vi "practiceImageAnalysis20vi.vi"() -> ()   [LabVIEW 2016]
uses:
  <vilib>/vision/Measure.llb/Straight Edge Options.ctl
  <vilib>/vision/Measure.llb/Straight Edge Process.ctl
  <vilib>/vision/Measure.llb/Edge Options.ctl
  <vilib>/vision/Measure.llb/Edge Polarity.ctl
  <vilib>/Analysis/6fits.llb/Curve Fitting Criteria.ctl
  <vilib>/Utility/file.llb/Write Delimited Spreadsheet (DBL).vi
  <vilib>/regexp/Match Regular Expression.xnode
  <vilib>/Analysis/NI_AALPro.lvlib
panel:
  in  "x values for fit line on plot":dbl[](array[numeric])=[-700.0, -300.0, 100.0, 500.0, 700.0]
  out "Bottom intercept":dbl
  out "Bottom slope":dbl
  out "Top intercept":dbl
  in  "method":T1 items=["Least Square", "Least Absolute Residual", "Bisquare"]
  out "Top slope":dbl
  out "Each point on located edges":T2(graph)
  out "Coordinate array for image capture":dbl[][](array[numeric])
  in  "Coordinate file for image capture":path=path "E:/XYZstage+Camera_CollectedImages/12-16-2016/noStaveMount/toolingpinsCoordinates-captured.csv"
  out "Review":bool
  out "Search running?":bool
  in  "Options: Bottom Edge Search":T5={"Search Direction"=3, "Edge Options"={"Edge Polarity"=2, "Kernel Size"=9, "Width"=3, "Minimum Edge Strength"=17.0, "Interpolation Type"=enum."Bilinear Fixed", "Data Processing Method"=enum."Average"}, "Show Search Area"=TRUE, "Show Search Lines"=TRUE, "Show Edges Found"=TRUE, "Show Result"=TRUE, "Search Area Color"=65280, "Search Lines Color"=255, "Edge Locations Color"=16776960, "Result Color"=16711680, "Overlay Group Name"=""} {"Search Direction" items=["Left to Right", "Right to Left", "Top to Bottom", "Bottom to Top"]; "Edge Options"."Edge Polarity" items=["All Edges", "Rising Edges", "Falling Edges"]; "Edge Options"."Minimum Edge Strength" format="%.2f"; "Edge Options"."Width" step=2; "Edge Options"."Kernel Size" step=2}
  in  "Options: Top Edge Search":T5={"Search Direction"=2, "Edge Options"={"Edge Polarity"=0, "Kernel Size"=5, "Width"=3, "Minimum Edge Strength"=16.0, "Interpolation Type"=enum."Bilinear Fixed", "Data Processing Method"=enum."Average"}, "Show Search Area"=TRUE, "Show Search Lines"=TRUE, "Show Edges Found"=TRUE, "Show Result"=TRUE, "Search Area Color"=65280, "Search Lines Color"=255, "Edge Locations Color"=16776960, "Result Color"=16711680, "Overlay Group Name"=""} {"Search Direction" items=["Left to Right", "Right to Left", "Top to Bottom", "Bottom to Top"]; "Edge Options"."Edge Polarity" items=["All Edges", "Rising Edges", "Falling Edges"]; "Edge Options"."Minimum Edge Strength" format="%.2f"; "Edge Options"."Width" step=2; "Edge Options"."Kernel Size" step=2}
  in  "Fit Options":T6={"Number of Lines"=1, "Type"=enum."First Edge Rake", "Min. Score"=10.0, "Max. Score"=1000.0, "Orientation"=0.0, "Angle Range"=45.0, "Angle Tolerance"=1.0, "Step Size"=196, "Min. SNR (db)"=0.0, "Min. Points (%)"=25.0, "Hough Iterations"=5} {"Min. Points (%)" min=0.0 max=100.0; "Min. SNR (db)" min=0.0; "Max. Score" min=0.0 max=1024.0; "Min. Score" min=0.0 max=1024.0 step=1.0}
  in  "Stop and delete":bool
  out "Images Array":T8[](array[plugin-control])
  in  "error in":errorcluster
  out "error out":errorcluster
  out "Filenames Array":string[](array[string])
  in  "Naming Convention":string="*.png"
  in  "Images Directory":path=path "E:/XYZstage+Camera_CollectedImages/12-16-2016/noStaveMount/toolingpins_images"
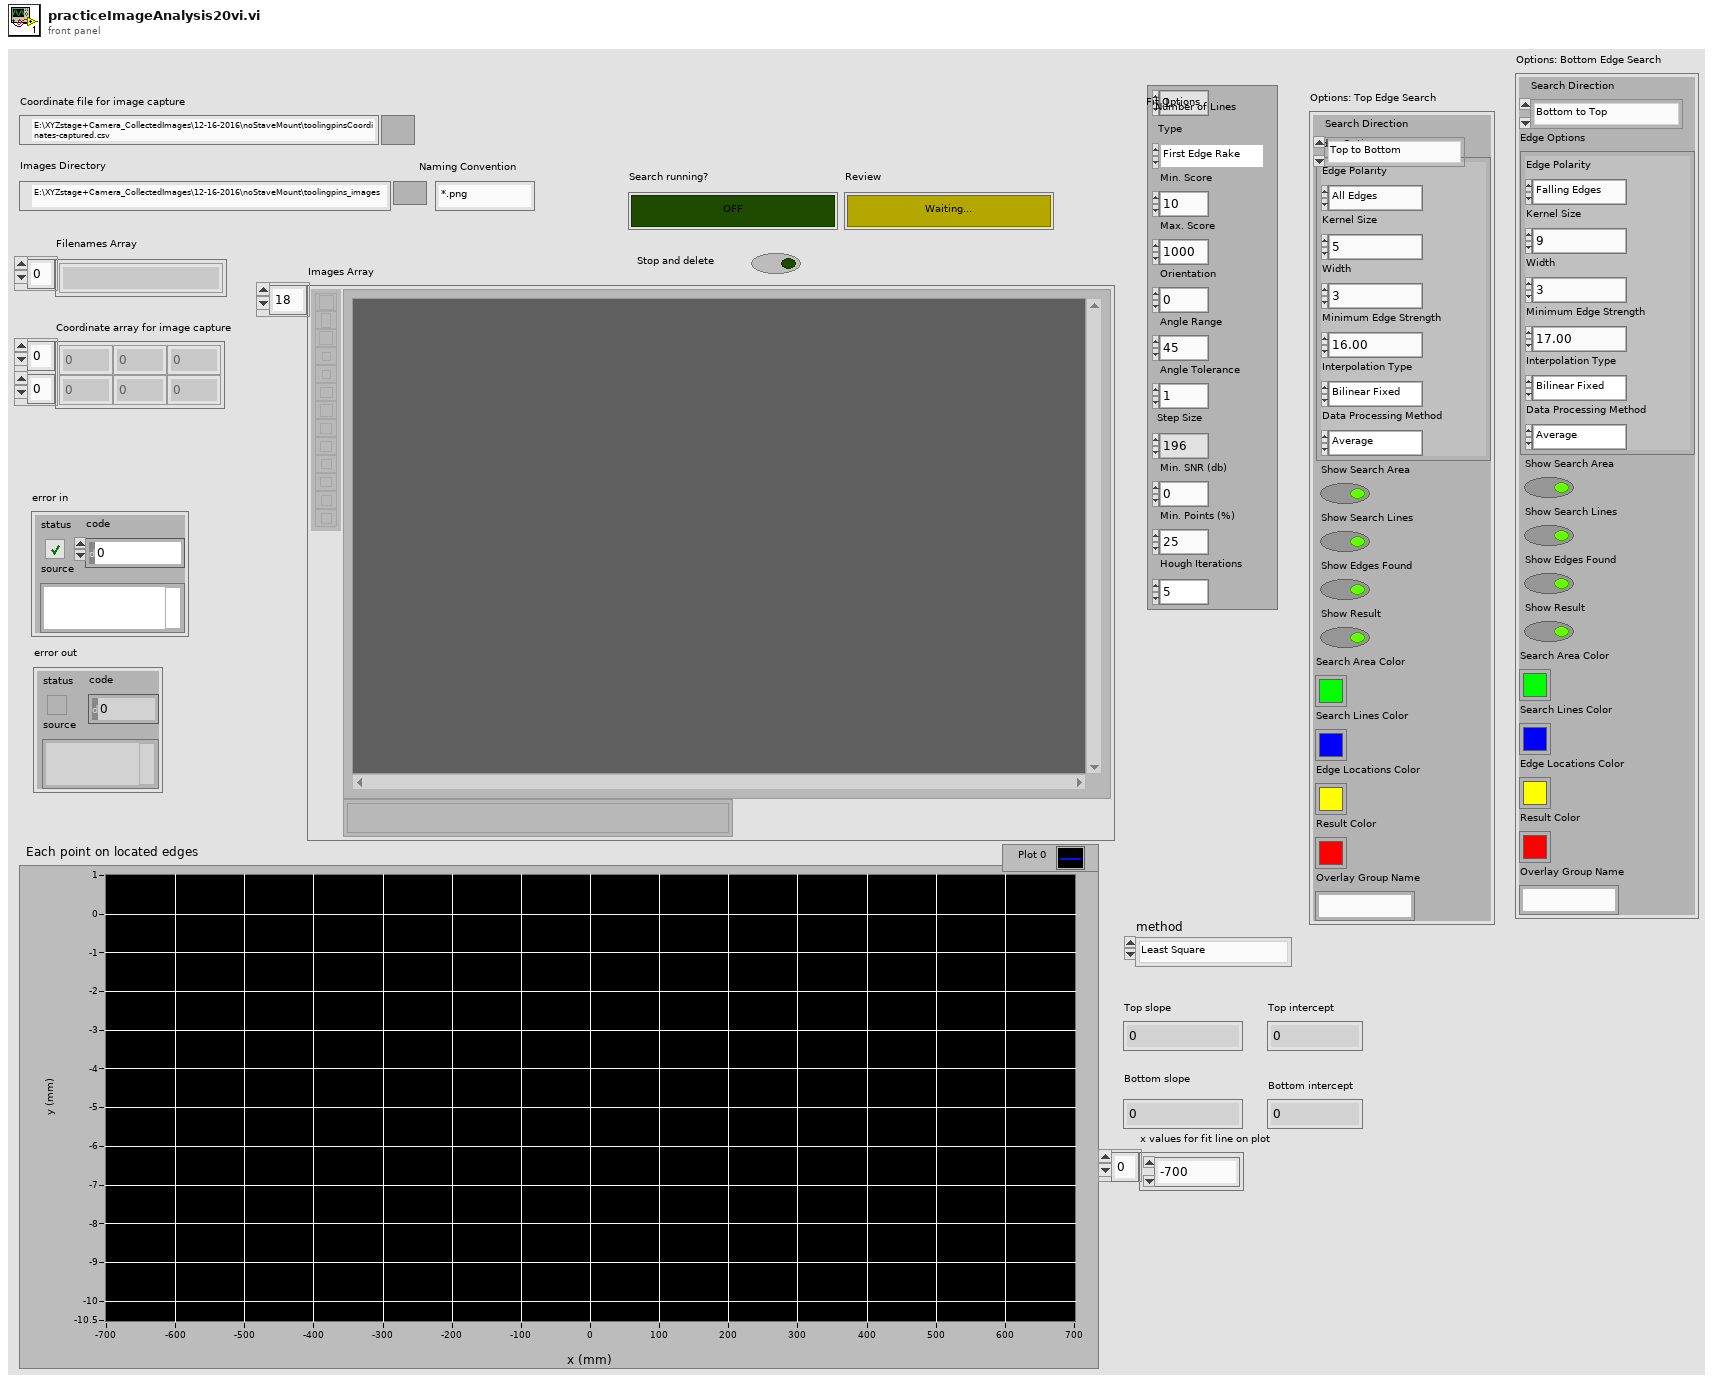
[diagram p1: front panel]
types:
  T1 = typedef "NI_AALPro.lvlib/Curve Fitting Criteria.ctl" = u16
  T2 = cluster{"Top averages":dbl[], "Best Linear Fit":dbl[]}[]
  T3 = typedef "Edge Options.ctl" = cluster{"Edge Polarity":T4, "Kernel Size":u32, "Width":u32, "Minimum Edge Strength":sgl, "Interpolation Type":enum32{"Zero Order", "Bilinear", "Quadratic", "Cubic", "Bilinear Fixed"}, "Data Processing Method":enum32{"Average", "Median"}}
  T4 = typedef "Edge Polarity.ctl" = u32
  T5 = cluster{"Search Direction":u32, "Edge Options":T3, "Show Search Area":bool, "Show Search Lines":bool, "Show Edges Found":bool, "Show Result":bool, "Search Area Color":u32, "Search Lines Color":u32, "Edge Locations Color":u32, "Result Color":u32, "Overlay Group Name":string}
  T6 = typedef "Straight Edge Options.ctl" = cluster{"Number of Lines":i32, "Type":T7, "Min. Score":dbl, "Max. Score":dbl, "Orientation":dbl, "Angle Range":dbl, "Angle Tolerance":dbl, "Step Size":u32, "Min. SNR (db)":dbl, "Min. Points (%)":dbl, "Hough Iterations":i32}
  T7 = typedef "Straight Edge Process.ctl" = enum32{"First Edge Rake", "Best Edge Rake", "Hough Edge Rake", "First Edge Projection", "Best Edge Projection"}
  T8 = typedef "IMAQ Image.ctl" = refnum<image>
  T9 = enum16{"cm", "mm", "pixels [mm/pix]", "pixels [um/pix]"}
  T10 = cluster{"Top averages":dbl[], "Top averages":dbl[]}
  T11 = cluster{"x values for fit line on plot":dbl[], "Array":dbl[]}
  T12 = cluster{"x values for fit line on plot":dbl[], "Array":dbl[]}[]
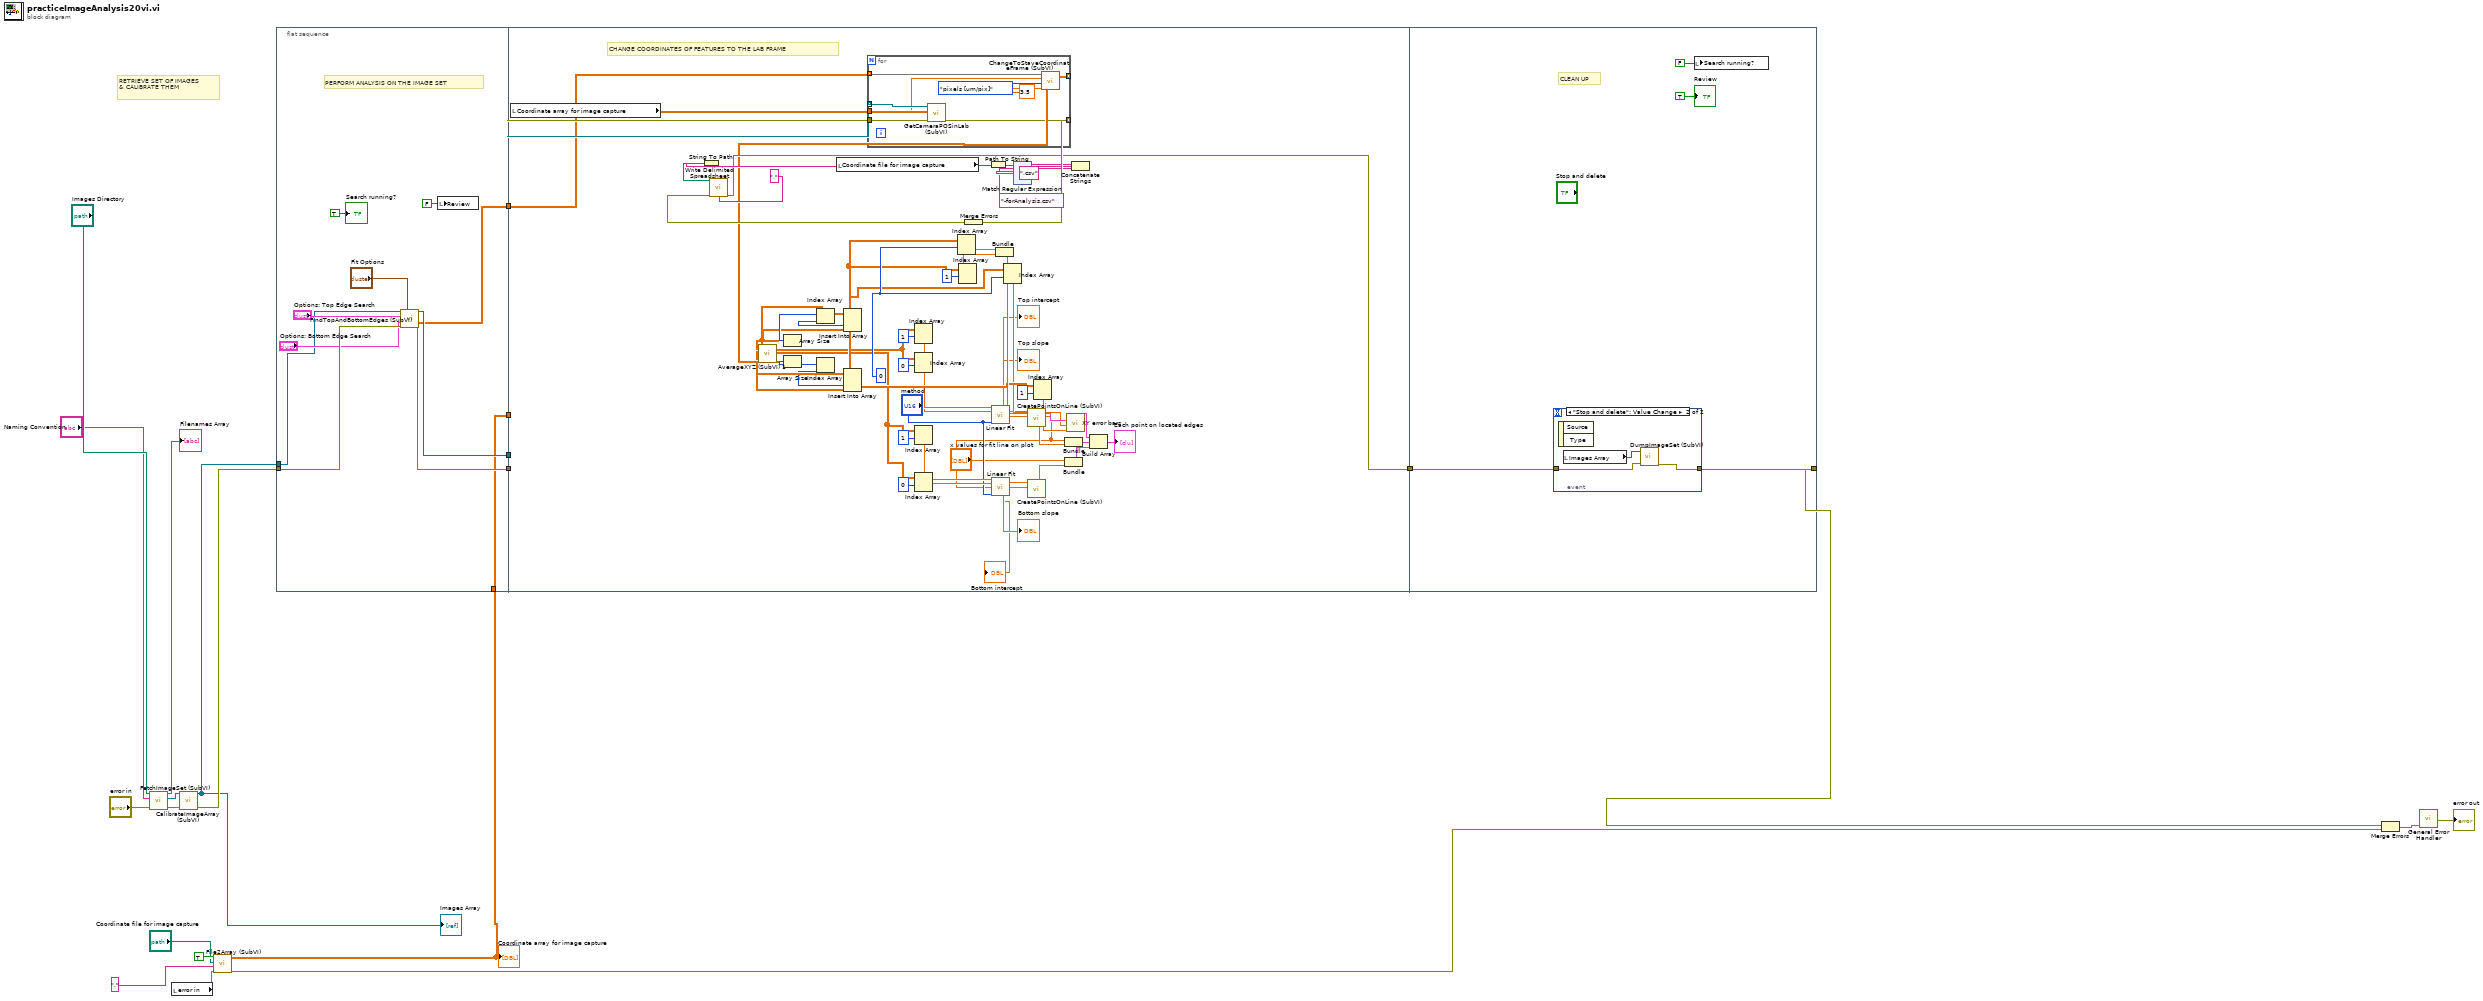
[diagram p0: block diagram]
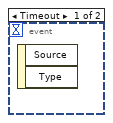
[diagram p2: hidden frame]
diagram:
  # "RETRIEVE SET OF IMAGES\n& CALIBRATE THEM"
  n1 = call "FetchImageSet (SubVI).vi"("error in (no error)"="error in", "Naming Convention"="Naming Convention", "Images Directory"="Images Directory") -> ("error out"=w18:errorcluster, "Image Array"=w19:T8[], "Filenames Array"=→"Filenames Array":string[])  [unwired: 6 in]
  n2 = local read "error in"() -> (w8:errorcluster)
  n3 = call "CalibrateImageArray (SubVI).vi"("error in (no error)"=w18, "Image Array"=w19) -> ("error out"=w15:errorcluster, "Calibrated Image Array"=w14:T8[])  [unwired: 7 in]
  "Images Array" <- w14
  n4 = call "File2Array (SubVI).vi"("error in (no error) in"=w8, "File delimiter"=",", "Source array file"="Coordinate file for image capture", "Load array from file?"=TRUE) -> ("error in (no error) out"=w6:errorcluster, "Loaded array"=w2:dbl[][])  [unwired: 6 in]
  "Coordinate array for image capture" <- w2
  n5 = flat-sequence {
    tunnel: w15 -> [w33]
    tunnel: w14 -> [w25]
    tunnel: [w32] -> w13
    tunnel: [w31] -> w12
    tunnel: [w24] -> w4
    tunnel: w2 -> [w23]
    tunnel: [w23] -> w1
    tunnel: w13 -> [w86]
    tunnel: w12 -> [w87]
    tunnel: w4 -> [w84]
    tunnel: [w73] -> w3
    tunnel: w1 -> [_]
    tunnel: [w212] -> w7
    tunnel: w3 -> [w211]
    frame #0 {
      # "PERFORM ANALYSIS ON THE IMAGE SET"
      n6 = call "FindTopAndBottomEdges (SubVI).vi"("Calibrated Image Array"=w25, "Fit Options"="Fit Options", "Options: Top Edge Search"="Options: Top Edge Search", "Options: Bottom Edge Search"="Options: Bottom Edge Search", "error in (no error)"=w33) -> ("Analyzed Image Array"=w31:T8[], "Array of Edge Endpoint Arrays"=w24:sgl[][][], "error out"=w32:errorcluster)  [unwired: 6 in, 2 out]
      n7 = local write "Review"(FALSE ("Review")) -> ()
      "Search running?" <- TRUE ("Search running?")
    }
    frame #1 {
      w70 = 0 ("index (row)")
      # "CHANGE COORDINATES OF FEATURES TO THE LAB FRAME"
      n8 = local read "Coordinate array for image capture"() -> (w85:dbl[][])
      n9 = local read "Coordinate file for image capture"() -> (w82:path)
      n10 = for {
        tunnel: w87 -> [w210] mode=indexing
        tunnel: w86 -> [w209]
        tunnel: w85 -> [w208]
        tunnel: w84 -> [w206] mode=indexing
        tunnel: [w203] -> w83 mode=indexing
        tunnel: [w202] -> w72 mode=indexing
        n11 = call "GetCameraPOSinLab (SubVI).vi"("error in (no error)"=w209, "Loaded array"=w208, "Refnum in"=w210) -> ("error out"=w203:errorcluster, "Image coordinates in lab frame"=w207:dbl[])  [unwired: 6 in, 1 out]
        n12 = call "ChangeToStaveCoordinateFrame (SubVI).vi"("Loaded array (image frame)"=w206, "Image Origin in XYZ Stage Coords [mm]"=w207, "Units"=T9."pixels [um/pix]", "Pixel resolution"=3.5) -> ("Array (stage frame, mm)"=w202:dbl[][])  [unwired: 2 in]
      }
      n13 = call "AverageXYZ (SubVI) 1.vi"("array"=w72) -> ("Bottom SD"=w63:dbl[][], "Bottom averages"=w47:dbl[][], "Top SD"=w66:dbl[][], "Top averages"=w52:dbl[][])  [unwired: 7 in]
      n14 = Array Size(array=w47) -> (size(s)=w69:i32[])
      n15 = Array Size(array=w63) -> (size(s)=w64:i32[])
      n16 = Index Array(array=w69) -> (element=w68:i32)  [unwired: 1 in]
      n17 = Index Array(array=w64) -> (element=w65:i32)  [unwired: 1 in]
      n18 = Insert Into Array(array=w52, index (col)=w68, new element=w47) -> (w67:dbl[][])  [unwired: 1 in]
      n19 = Insert Into Array(array=w66, index (col)=w65, new element=w63) -> (w61:dbl[][])  [unwired: 1 in]
      n20 = Index Array(array=w52, index (row)=1) -> (element=w54:dbl[])  [unwired: 1 in]
      n21 = Index Array(array=w52, index (row)=0) -> (element=w53:dbl[])  [unwired: 1 in]
      n22 = Index Array(array=w47, index (row)=1) -> (element=w49:dbl[])  [unwired: 1 in]
      n23 = Index Array(array=w47, index (row)=0) -> (element=w48:dbl[])  [unwired: 1 in]
      n24 = Index Array(array=w67, index (row)=w70) -> (element=w45:dbl[])  [unwired: 1 in]
      n25 = Index Array(array=w67, index (row)=1) -> (element=w57:dbl[])  [unwired: 1 in]
      n26 = Merge Errors(w83) -> (w74:errorcluster)
      n27 = Path To String(path=w82) -> (string=w80:string)
      n28 = call <vilib>:"Linear Fit.vi"("Y"=w54, "X"=w53, "method"="method") -> ("slope"=w42:dbl, "intercept"=w41:dbl)  [unwired: 8 in, 3 out]
      "Top slope" <- w42
      "Top intercept" <- w41
      n29 = call <vilib>:"Linear Fit.vi"("Y"=w49, "X"=w48, "method"="method") -> ("slope"=w38:dbl, "intercept"=w37:dbl)  [unwired: 8 in, 3 out]
      "Bottom slope" <- w38
      "Bottom intercept" <- w37
      n30 = Bundle("Top averages"=w45, "Top averages"=w57) -> (w62:T10)  [unwired: 1 in]
      n31 = Index Array(array=w61, index (row)=w70) -> (element=w59:dbl[])  [unwired: 1 in]
      n32 = xnode "Match Regular Expression"("input string"=w80, "regular expression"=".csv") -> ("before match"=w78:string)  [unwired: 4 in, 4 out]
      n33 = call "CreatePointsOnLine (SubVI).vi"("x values for fit line on plot"="x values for fit line on plot", "intercept"=w41, "slope"=w42) -> ("Array"=w40:dbl[])  [unwired: 8 in]
      n34 = call "CreatePointsOnLine (SubVI).vi"("x values for fit line on plot"="x values for fit line on plot", "intercept"=w37, "slope"=w38) -> ("Array"=w39:dbl[])  [unwired: 8 in]
      n35 = Index Array(array=w61, index (row)=1) -> (element=w58:dbl[])  [unwired: 1 in]
      n36 = Bundle("x values for fit line on plot"="x values for fit line on plot", "Array"=w40) -> (w35:T11)  [unwired: 1 in]
      n37 = Bundle("x values for fit line on plot"="x values for fit line on plot", "Array"=w39) -> (w36:T11)  [unwired: 1 in]
      n38 = call "XY error bars.vi"("XY plot"=w62, "Xerror"=w59, "Yerror"=w58) -> ("X+Y error bars"=w44:cluster{dbl[], dbl[]})  [unwired: 5 in, 2 out]
      n39 = Concatenate Strings(w78, "-forAnalysis.csv" ("name or relative path")) -> (w77:string)
      n40 = String To Path(string=w77) -> (path=w75:path)
      n41 = call-poly <vilib>:"Write Delimited Spreadsheet.vi"("file path (dialog if empty)"=w75, "error in (no error)"=w74, "delimiter (\\t)"="," ("delimiter (\\t)")) -> ("error out"=w73:errorcluster)  [unwired: 11 in, 1 out]
      n42 = Build Array(w44, w35, w36) -> (→"Each point on located edges":T12)
    }
    frame #2 {
      # "CLEAN UP"
      n43 = event shown="[1] \"Stop and delete\": Value Change" {
        selector: _ -> [_ _]
        dyn-events: _ -> [_ _]
        timeout: _ -> [_ _]
        tunnel: [_ w217] -> w212
        tunnel: w211 -> [_ w216]
        event Timeout {
          n44 = event-data() -> ()  [unwired: 1 in, 2 out]
        }
        event "Stop and delete": Value Change {
          n45 = event-data() -> ()  [unwired: 1 in, 2 out]
          n46 = local read "Images Array"() -> (w215:T8[])
          n47 = call "DumpImageSet (SubVI).vi"("error in (no error)"=w216, "Calibrated Image Array"=w215) -> ("error out"=w217:errorcluster)  [unwired: 6 in]
        }
      }
      n48 = local write "Search running?"(FALSE ("Search running?")) -> ()
      "Review" <- TRUE ("Review")
    }
  }
  n49 = Merge Errors(w7, w6) -> (w5:errorcluster)
  n50 = call <vilib>:"General Error Handler.vi"("error in (no error)"=w5) -> ("error out"=→"error out":errorcluster)  [unwired: 10 in, 4 out]
